vi "ReadExecutableConfiguration.vi"(8 "Error In":errorcluster, 11 "VI Path":path) -> (0 "Error Out":errorcluster, 3 "Executable Configuration":T1)   [LabVIEW 2012]
uses:
  ExecutableConfiguration.ctl
  <vilib>/Utility/config.llb/Read Key (Path).vi
  <vilib>/Utility/config.llb/Read Key (I32).vi
  <vilib>/Utility/config.llb/Read Key (Boolean).vi
  <vilib>/Utility/config.llb/NI_LVConfig.lvlib
  libs/LV-Utilities/LV-Utilities.lvlib
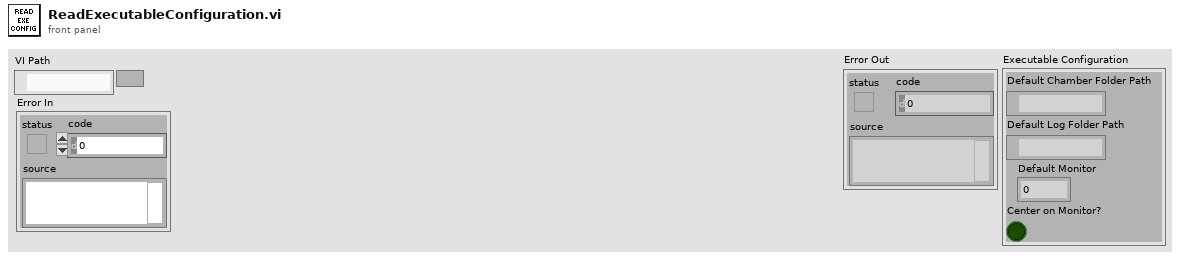
[diagram p1: front panel]
types:
  T1 = typedef "ExecutableConfiguration.ctl" = cluster{"Default Chamber Folder Path":path, "Default Log Folder Path":path, "Default Monitor":i32, "Center on Monitor?":bool}
  T2 = typedef "NI_LVConfig.lvlib/Config Data RefNum.ctl" = refnum<k1>
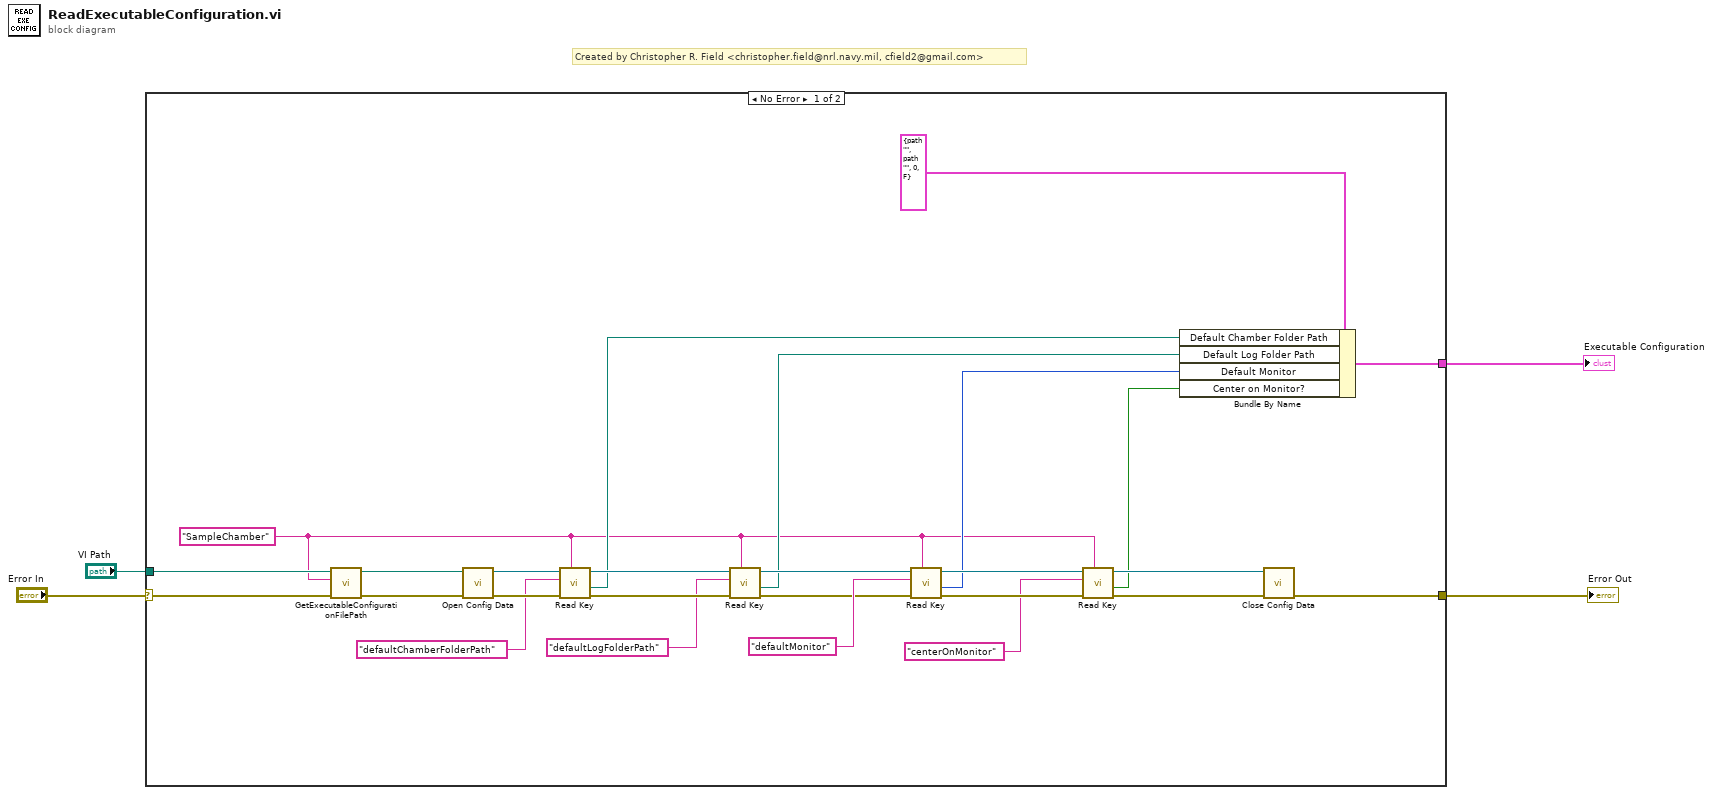
[diagram p0: block diagram]
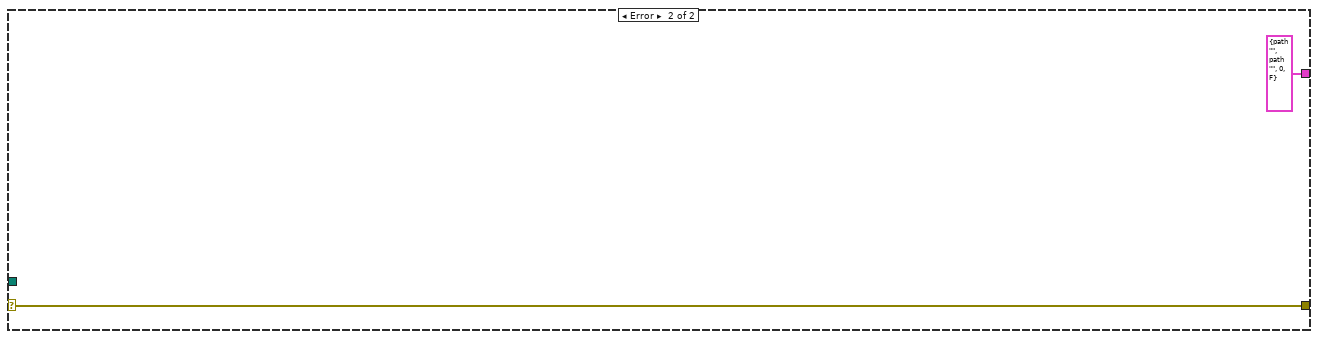
[diagram p2: hidden frame]
diagram:
  # "Created by Christopher R. Field <christopher.field@nrl.navy.mil, cfield2@gmail.com>"
  n1 = case shown="No Error" "Error In" {
    selector: "Error In" -> [w5 w32]
    tunnel: [w26 w32] -> w4
    tunnel: [w10 T1 {"Default Chamber Folder Path"=path "", "Default Log Folder Path"=path "", "Default Monitor"=0, "Center on Monitor?"=FALSE} ("Executable Configuration")] -> w3
    tunnel: "VI Path" -> [w7 _]
    frame No Error {
      w6 = "SampleChamber" ("section")
      n2 = call "GetExecutableConfigurationFilePath.vi"("Error In"=w5, "Application Name"=w6, "VI Path"=w7) -> ("Error Out"=w9:errorcluster, "Executable Config File Path"=w8:path)  [unwired: 7 in]
      n3 = call <vilib>:"Open Config Data.vi"("error in (no error)"=w9, "configuration file path"=w8) -> ("error out"=w29:errorcluster, "refnum"=w30:T2)  [unwired: 7 in, 1 out]
      n4 = call-poly <vilib>:"Read Key.vi"("section"=w6, "error in (no error)"=w29, "key"="defaultChamberFolderPath", "refnum"=w30) -> ("error out"=w19:errorcluster, "value"=w14:path, "refnum out"=w20:T2)  [unwired: 4 in, 1 out]
      n5 = call-poly <vilib>:"Read Key.vi"("section"=w6, "error in (no error)"=w19, "key"="defaultLogFolderPath", "refnum"=w20) -> ("error out"=w17:errorcluster, "value"=w13:path, "refnum out"=w18:T2)  [unwired: 4 in, 1 out]
      n6 = call-poly <vilib>:"Read Key.vi"("section"=w6, "error in (no error)"=w17, "key"="defaultMonitor", "refnum"=w18) -> ("error out"=w24:errorcluster, "value"=w12:i32, "refnum out"=w25:T2)  [unwired: 4 in, 1 out]
      n7 = call-poly <vilib>:"Read Key.vi"("section"=w6, "error in (no error)"=w24, "key"="centerOnMonitor", "refnum"=w25) -> ("error out"=w23:errorcluster, "value"=w11:bool, "refnum out"=w22:T2)  [unwired: 4 in, 1 out]
      n8 = Bundle By Name(cluster=T1 {"Default Chamber Folder Path"=path "", "Default Log Folder Path"=path "", "Default Monitor"=0, "Center on Monitor?"=FALSE} ("Executable Configuration"), "Default Chamber Folder Path"=w14, "Default Log Folder Path"=w13, "Default Monitor"=w12, "Center on Monitor?"=w11) -> (w10:T1)
      n9 = call <vilib>:"Close Config Data.vi"("error in (no error)"=w23, "refnum"=w22) -> ("error out"=w26:errorcluster)  [unwired: 8 in, 1 out]
    }
    frame Error {
    }
  }
  "Error Out" <- w4
  "Executable Configuration" <- w3
